vi "Read_Packet_from_TDMS.vi"(8 "error in (no error)":errorcluster, 11 "TDMS File path":path) -> (0 "error out":errorcluster, 2 "Total Frame Num":i32, 3 "Line Packet Payload":u8[][](array[numeric]))   [LabVIEW 2020]
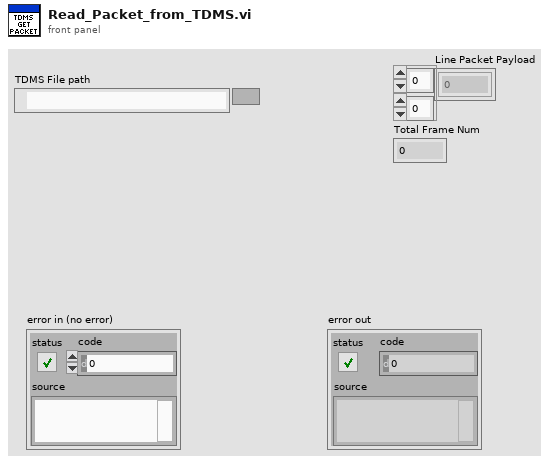
[diagram p1: front panel]
types:
  T1 = enum16{"open", "open or create", "create or replace", "create", "open (read-only)"}
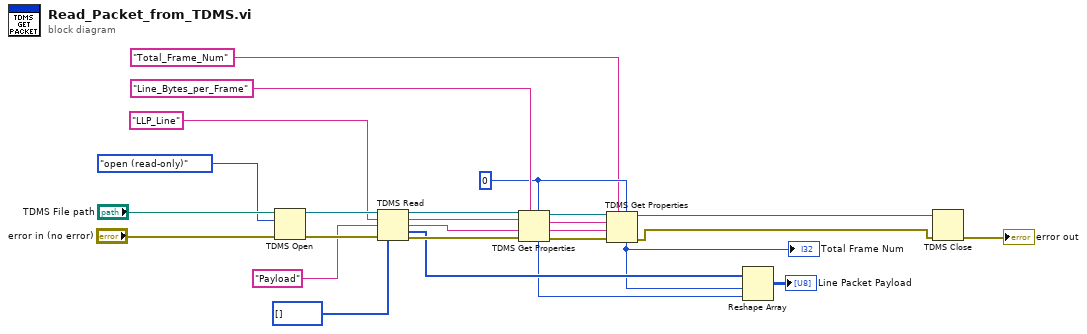
[diagram p0: block diagram]
diagram:
  w8 = 0
  n1 = TDMS Open(8:"error in (no error)", 10:T1."open (read-only)" ("operation (0:open)"), 11:"TDMS File path") -> (0:w22:errorcluster, 3:w23:refnum<k34>)  [unwired: 4 in]
  n2 = TDMS Read(0:w23, 5:"LLP_Line" ("Save to Group"), 7:"Payload" ("channel name"), 11:w22, 12:u8[] []) -> (4:w17:refnum<k34>, 6:w15:string, 8:w14:string, 10:w6:u8[], 15:w16:errorcluster)  [unwired: 3 in, 1 out]
  n3 = TDMS Get Properties(5:w8, 7:"Line_Bytes_per_Frame", 8:w16, 9:w14, 10:w15, 11:w17) -> (0:w9:errorcluster, 1:w10:string, 2:w11:string, 3:w12:refnum<k34>, 4:w4:i32)  [unwired: 1 out]
  n4 = TDMS Get Properties(5:w8, 7:"Total_Frame_Num", 8:w9, 9:w10, 10:w11, 11:w12) -> (0:w1:errorcluster, 3:w2:refnum<k34>, 4:w5:i32)  [unwired: 3 out]
  "Total Frame Num" <- w5
  n5 = Reshape Array(w6, w5, w4) -> (→"Line Packet Payload":u8[][])
  n6 = TDMS Close(8:w1, 11:w2) -> (0:→"error out":errorcluster)  [unwired: 1 out]
